vi "Gear On.vi"(8 "error in":errorcluster) -> (0 "error out":errorcluster)   [LabVIEW 2016, in "Intake.lvlib"]
uses:
  Intake.lvlib
  Typedef/Intake Command.ctl
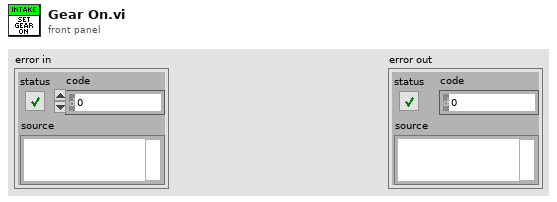
[diagram p1: front panel]
types:
  T1 = typedef "Intake.lvlib/Intake Command.ctl" = enum16{"Gear On", "Gear Off", "Gear Reverse", "Gear Release", "Fuel Deploy", "Fuel Retract", "Fuel Agitate", "Fuel Reverse"}
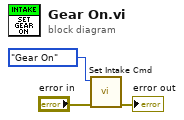
[diagram p0: block diagram]
diagram:
  n1 = call "Set Intake Cmd.vi"("error in"="error in", "Cmd"=Intake_Command."Gear On") -> ("error out"=→"error out":errorcluster)  [unwired: 9 in]
